vi "Sensors and valves.vi"() -> ()   [LabVIEW 2021]
uses:
  Classes/Controller/I-O/I-O.lvclass
  Classes/Controller/Controller.lvclass
panel:
  in  "2":bool
  in  "?":bool
  in  "?":bool[](array[boolean])
  in  "?":bool[](array[boolean])
  in  "?":bool[](array[boolean])
  out "Compression Sensor":bool[](array[boolean])
  out "Tool Secondary Sensor":bool[](array[boolean])
  out "Tool Primary Sensor":bool[](array[boolean])
  out "Region Sensors":bool[](array[boolean])
  out "Positions Region 2":bool[](array[boolean])
  out "Positions Region 1":bool[](array[boolean])
  in  "Stop":bool
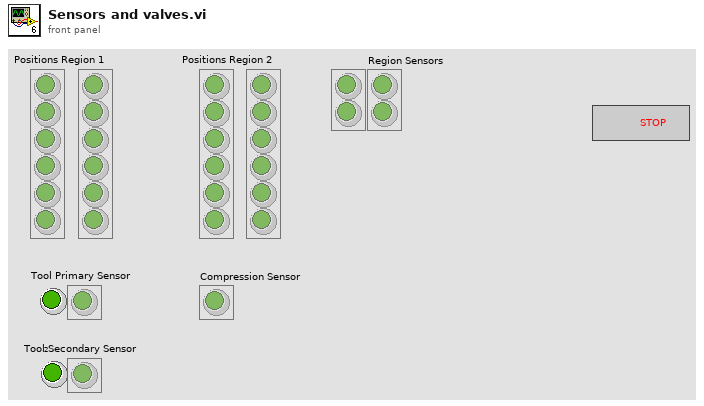
[diagram p1: front panel]
types:
  T1 = typedef "Controller.lvclass/Controllers.ctl" = cluster{"I-O.lvclass":refnum<class "I-O.lvclass">, "Gantry":refnum<k24>, "Dispenser":refnum<visa-resource-name>}
  T2 = typedef "I-O.lvclass/Pin Map.ctl" = cluster{"Region Valves":i32[], "Extra Valves":dbl[][][], "Tool Primary Valve":i32, "Tool Secondary Valve":i32, "Region Sensors":i32[], "Extra Sensors":dbl[][][], "Tool Primary Sensor":dbl, "Tool Secondary Sensor":dbl, "Compression Sensor":dbl, "5V":i32, "Dispenser Sensor":dbl}
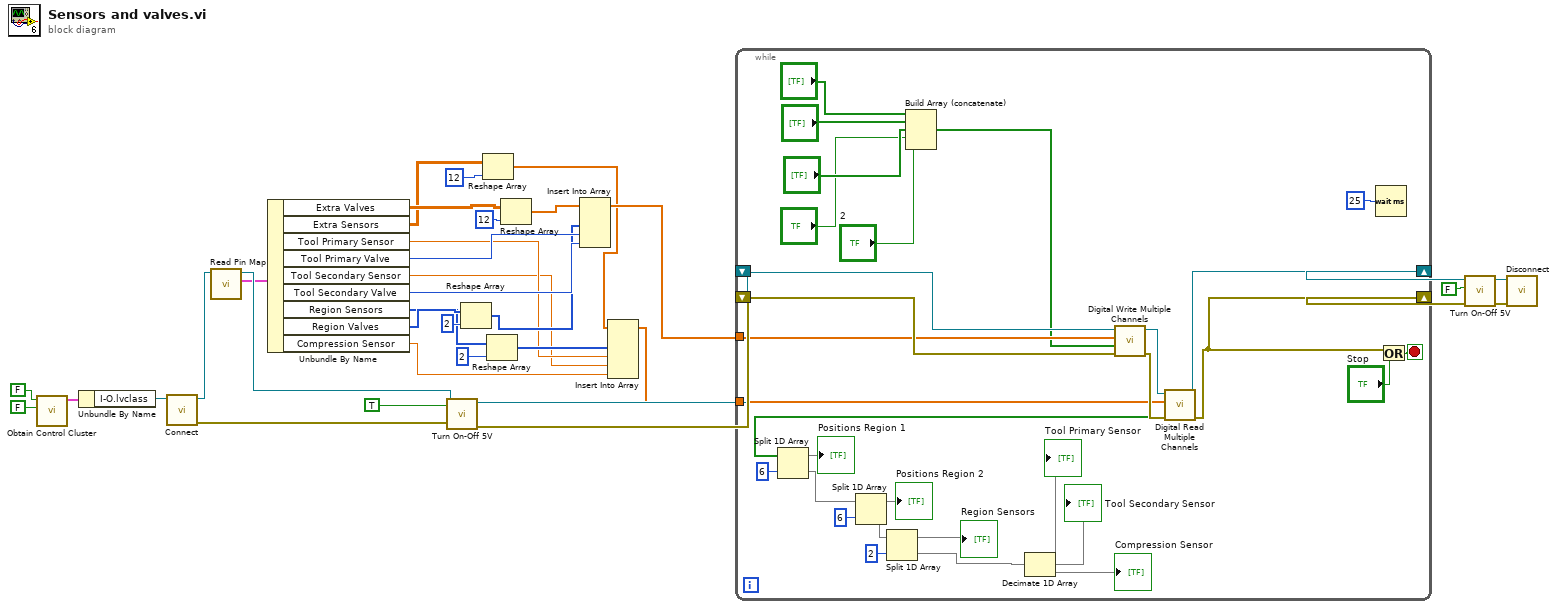
[diagram p0: block diagram]
diagram:
  n1 = call "Obtain Control Cluster.vi"("Dispense"=FALSE, "Motion"=FALSE) -> ("Control Out"=w34:T1)  [unwired: 9 in]
  n2 = Unbundle By Name(w34) -> ("I-O.lvclass"=w35:refnum<class "I-O.lvclass">)
  n3 = call-dynamic "Connect.vi"("Controller in"=w35) -> ("error out"=w28:errorcluster, "Controller out"=w27:refnum<class "I-O.lvclass">)  [unwired: 9 in]
  n4 = call-dynamic "Read Pin Map.vi"("I-O in"=w27) -> ("Pin Map 2"=w25:T2, "I-O out"=w26:refnum<class "I-O.lvclass">)  [unwired: 8 in, 1 out]
  n5 = Unbundle By Name(w25) -> ("Extra Valves"=w16:dbl[][][], "Extra Sensors"=w7:dbl[][][], "Tool Primary Sensor"=w4:dbl, "Tool Primary Valve"=w14:i32, "Tool Secondary Sensor"=w3:dbl, "Tool Secondary Valve"=w15:i32, "Region Sensors"=w9:i32[], "Region Valves"=w11:i32[], "Compression Sensor"=w2:dbl)
  n6 = call-dynamic "Turn On-Off 5V.vi"("error in (no error)"=w28, "Value"=TRUE, "I-O in"=w26) -> ("error out"=w29:errorcluster, "I-O out"=w20:refnum<class "I-O.lvclass">)  [unwired: 7 in]
  n7 = Reshape Array(w11, 2 ("dimension size")) -> (w10:i32[])
  n8 = Reshape Array(w7, 12 ("dimension size")) -> (w6:dbl[])
  n9 = Reshape Array(w9, 2 ("dimension size")) -> (w5:i32[])
  n10 = Reshape Array(w16, 12 ("dimension size")) -> (w17:dbl[])
  n11 = Insert Into Array(array=w17, new element #1=w10, new element #2=w14, new element #3=w15) -> (w8:dbl[])  [unwired: 1 in]
  n12 = Insert Into Array(array=w6, new element #1=w5, new element #2=w4, new element #3=w3, new element #4=w2) -> (w1:dbl[])  [unwired: 1 in]
  n13 = while {
    shift-right: [w57] -> w23
    shift-left: w20 -> [w62]
    shift-right: [w58] -> w30
    shift-left: w29 -> [w61]
    tunnel: w8 -> [w56]
    tunnel: w1 -> [w55]
    stop <- w63 stop-if-true
    n14 = Build Array (concatenate)("?", "?", "?", "?", "2") -> (w36:bool[])
    n15 = call-dynamic "Digital Write Multiple Channels.vi"("error in (no error)"=w61, "values"=w36, "indices"=w56, "I-O in"=w62) -> ("error out"=w60:errorcluster, "I-O out"=w59:refnum<class "I-O.lvclass">)  [unwired: 6 in]
    n16 = call-dynamic "Digital Read Multiple Channels.vi"("error in (no error)"=w60, "indices"=w55, "I-O in"=w59) -> ("error out"=w58:errorcluster, "Array 2"=w54:bool[], "I-O out"=w57:refnum<class "I-O.lvclass">)  [unwired: 6 in]
    n17 = Split 1D Array(array=w54, index=6) -> (first subarray=→"Positions Region 1":bool[], second subarray=w50:bool[])
    n18 = Split 1D Array(array=w50, index=6) -> (first subarray=→"Positions Region 2":bool[], second subarray=w47:bool[])
    n19 = Split 1D Array(array=w47, index=2) -> (first subarray=→"Region Sensors":bool[], second subarray=w45:bool[])
    n20 = Decimate 1D Array(w45) -> (→"Tool Primary Sensor":bool[], →"Tool Secondary Sensor":bool[], →"Compression Sensor":bool[])
    n21 = Wait (ms)(milliseconds to wait=u32 25) -> ()  [unwired: 1 out]
    n22 = Or(x=w58, y="Stop") -> (x .or. y?=w63:bool)
  }
  n23 = call-dynamic "Turn On-Off 5V.vi"("error in (no error)"=w30, "Value"=FALSE, "I-O in"=w23) -> ("error out"=w31:errorcluster, "I-O out"=w22:refnum<class "I-O.lvclass">)  [unwired: 7 in]
  n24 = call-dynamic "Disconnect.vi"("error in (no error)"=w31, "I-O in"=w22) -> ()  [unwired: 8 in, 1 out]
